vi "Clean up Auto scripting.vi"(11 "Programs":string[](array[string])) -> (3 "Array":string[](array[string]))   [LabVIEW 2013]
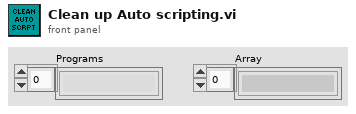
[diagram p1: front panel]
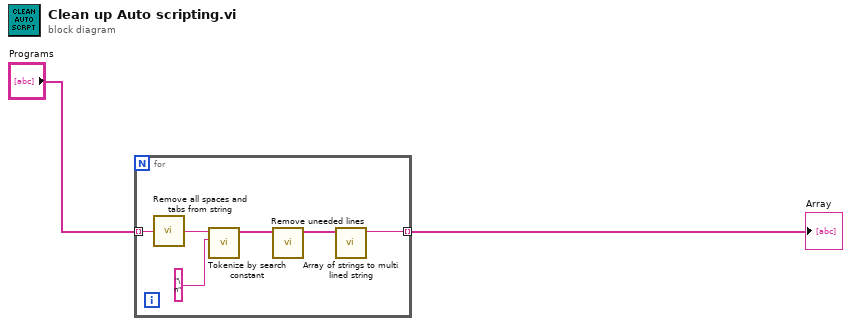
[diagram p0: block diagram]
diagram:
  n1 = for {
    tunnel: "Programs" -> [w7] mode=indexing
    tunnel: [w5] -> w2 mode=indexing
    n2 = call "Remove all spaces and tabs from string.vi"("String in"=w7) -> ("String out"=w6:string)
    n3 = call "Tokenize by search constant.vi"("search constant"="\n", "Data"=w6) -> ("Array"=w8:string[])  [unwired: 9 in]
    n4 = call "Remove uneeded lines.vi"("Array"=w8) -> ("Array out"=w3:string[])  [unwired: 10 in]
    n5 = call "Array of strings to multi lined string.vi"("Array in"=w3) -> ("Program"=w5:string)  [unwired: 10 in]
  }
  "Array" <- w2
